vi "Write Log File.vi"(6 "time":dbl format="%.3fs", 7 "error? (F)":bool, 8 "error in (no error)":errorcluster, 9 "line text":string, 10 "line tag":string, 11 "file refnum in":refnum<file>) -> (0 "error out":errorcluster, 3 "file refnum out":refnum<file>)   [LabVIEW 2021, in "DSF Core.lvlib" / "Logging Thread.lvclass"]
uses:
  Logging Thread.lvclass
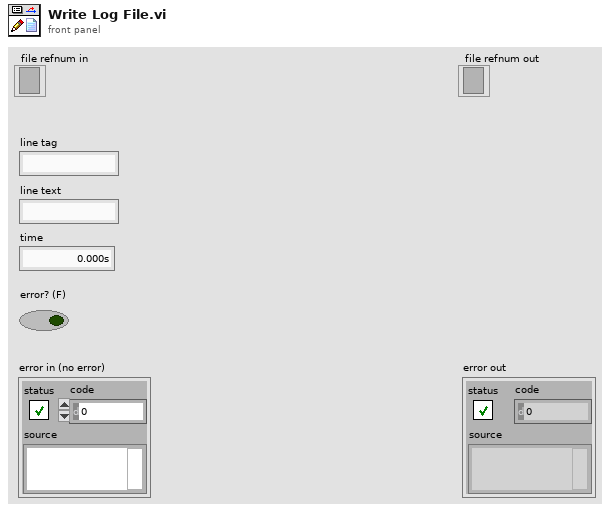
[diagram p1: front panel]
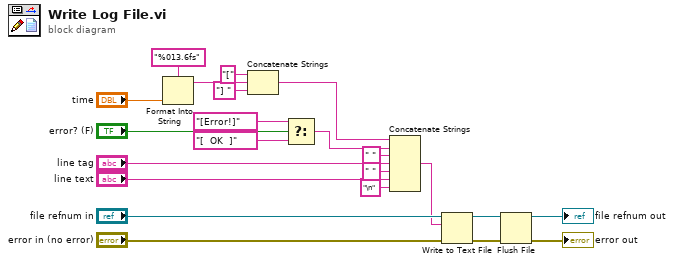
[diagram p0: block diagram]
diagram:
  n1 = Format Into String(format string="%013.6fs", "time") -> (resulting string=w11:string)  [unwired: 2 in, 1 out]
  n2 = Concatenate Strings("[" ("string"), w11, "] " ("string")) -> (w7:string)
  n3 = Select(t="[Error!]", s="error? (F)", f="[  OK  ]") -> (s? t:f=w6:string)
  n4 = Concatenate Strings(w7, w6, " " ("string"), "line tag", " " ("string"), "line text", "\n" ("string")) -> (w20:string)
  n5 = Write to Text File(file (use dialog)="file refnum in", text=w20, error in="error in (no error)") -> (refnum out=w4:refnum<file>, error out=w2:errorcluster)  [unwired: 1 in, 1 out]
  n6 = Flush File(refnum=w4, error in=w2) -> (refnum out=→"file refnum out":refnum<file>, error out=→"error out":errorcluster)
